vi "Add Configuration Files Section.vi"(8 "error in":errorcluster, 11 "Custom device Ref":T1 format="%.0x") -> (0 "error out":errorcluster, 2 "Configuration files Ref":T1 format="%.0x", 3 "Custom device Ref out":T1 format="%.0x")   [LabVIEW 2020, in "AIM ARINC 429 Scripting.lvlib"]
uses:
  AIM ARINC 429 Scripting.lvlib
  <vilib>/NI VeriStand/Custom Device API/Custom Device Item Ref.ctl
  Constants.vi
  <vilib>/NI VeriStand/Custom Device API/Custom Device API.lvlib
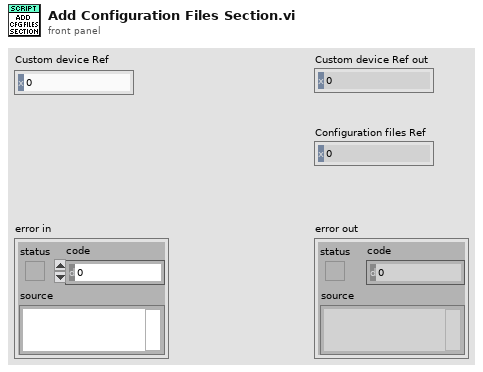
[diagram p1: front panel]
types:
  T1 = typedef "Custom Device API.lvlib/Custom Device Item Ref.ctl" = u64
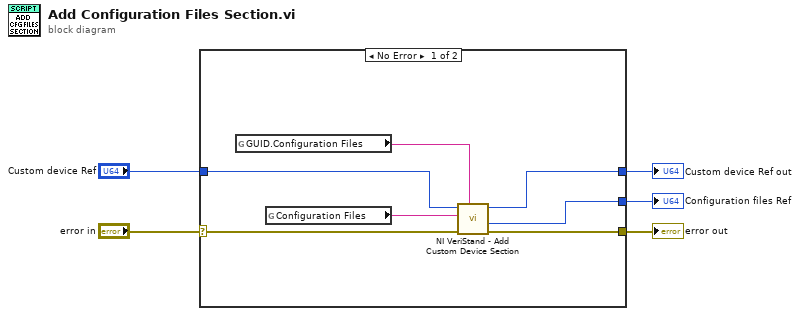
[diagram p0: block diagram]
diagram:
  n1 = case shown="No Error" "error in" {
    selector: "error in" -> [w10 w14]
    tunnel: "Custom device Ref" -> [w11 w13]
    tunnel: [w12 w14] -> w4
    tunnel: [w9 w13] -> w2
    tunnel: [w6 _] -> w1
    frame No Error {
      n2 = global read "Constants.vi" "GUID.Configuration Files"() -> (w7:string)
      n3 = global read "Constants.vi" "Configuration Files"() -> (w8:string)
      n4 = call <vilib>:"NI VeriStand - Add Custom Device Section.vi"("GUID (Default Section)"=w7, "error in (no error)"=w10, "Section Name"=w8, "Parent Ref in"=w11) -> ("error out"=w12:errorcluster, "Section Ptr"=w6:T1, "Parent Ref out"=w9:T1)  [unwired: 4 in, 1 out]
    }
    frame Error {
    }
  }
  "error out" <- w4
  "Custom device Ref out" <- w2
  "Configuration files Ref" <- w1
